vi "menuBarSelection.vi"(8 "error in (no error)":errorcluster, 10 "itemPath":string, 11 "ScriptEditorV2 in":refnum<class "ScriptEditorV2.lvclass">) -> (0 "error out":errorcluster, 2 "close":bool, 3 "ScriptEditorV2 out":refnum<class "ScriptEditorV2.lvclass">)   [LabVIEW 2009, in "Views.lvlib" / "ScriptEditor.lvlib" / "ScriptEditorV2.lvclass"]
uses:
  ScriptEditorV2.lvclass
  ScriptEditorV2.lvclass/ScriptEditorV2.ctl
  Tools/DatabaseHelpers.lvlib
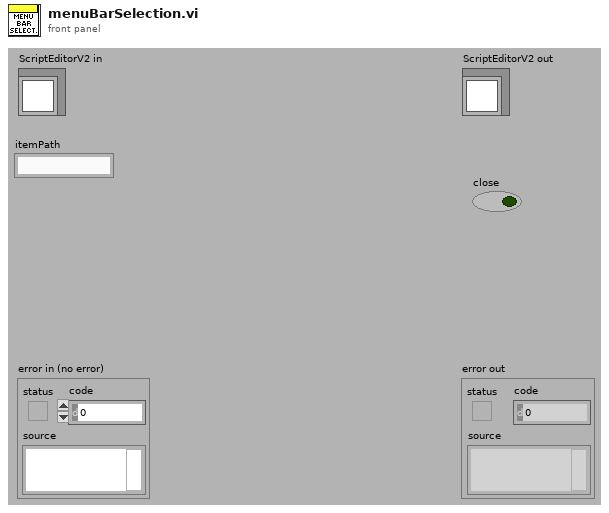
[diagram p1: front panel]
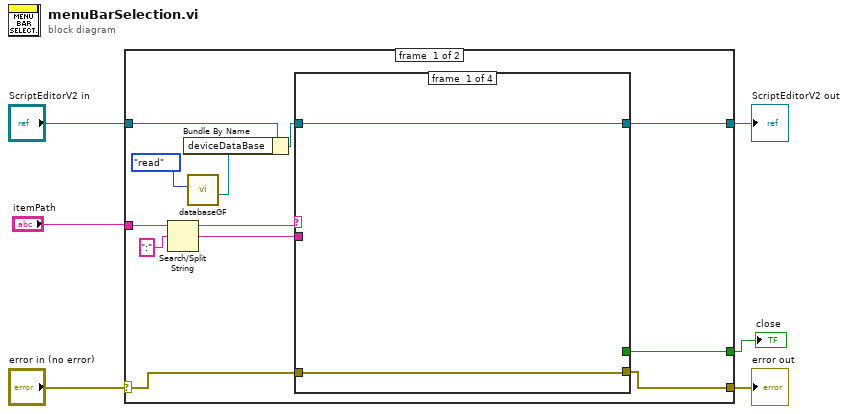
[diagram p0: block diagram]
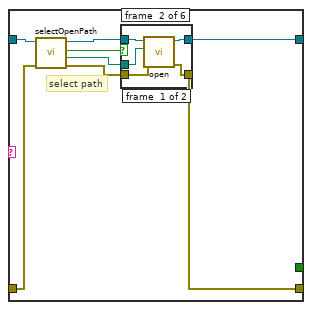
[diagram p3: hidden frame]
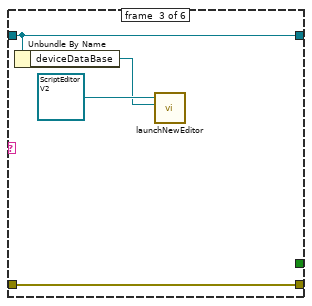
[diagram p5: hidden frame]
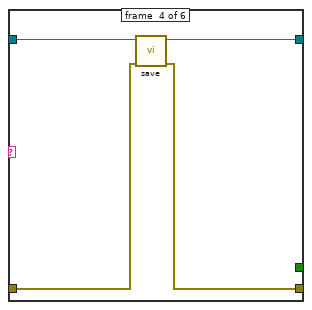
[diagram p6: hidden frame]
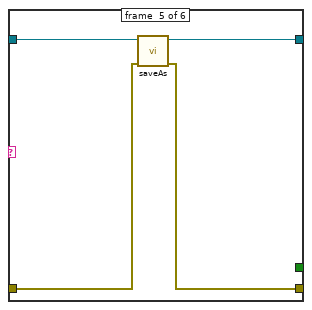
[diagram p7: hidden frame]
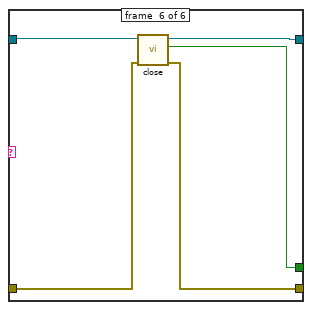
[diagram p8: hidden frame]
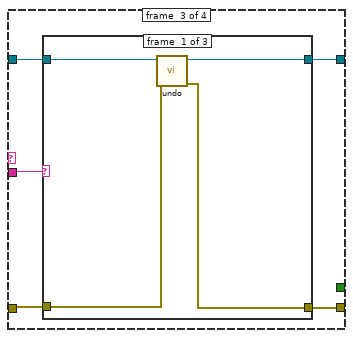
[diagram p9: hidden frame]
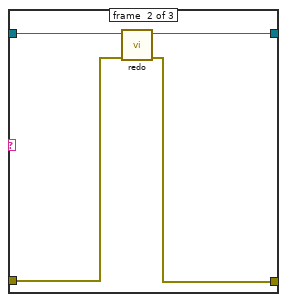
[diagram p10: hidden frame]
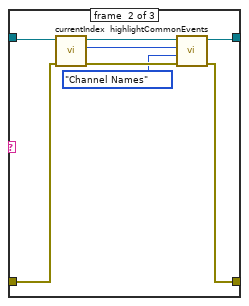
[diagram p13: hidden frame]
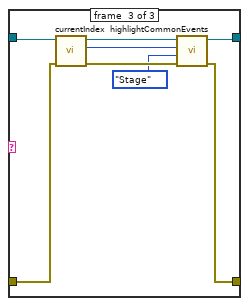
[diagram p14: hidden frame]
diagram:
  n1 = case shown="No Error" "error in (no error)" {
    selector: "error in (no error)" -> [w16 w100]
    tunnel: [w15 w100] -> w5
    tunnel: [w12 w99] -> w3
    tunnel: "ScriptEditorV2 in" -> [w8 w99]
    tunnel: "itemPath" -> [w17 _]
    tunnel: [w11 _] -> w1
    frame #0 {
      n2 = Search/Split String(string=w17, search string/char (-)=":") -> (substring before match=w14:string, match + rest of string=w13:string)  [unwired: 1 in, 1 out]
      n3 = call "databaseGF.vi"("Enum"=enum16{"write", "read"}."read") -> ("deviceDataBase out"=w9:refnum<class "deviceDataBase.lvclass">)  [unwired: 10 in]
      n4 = Bundle By Name(cluster=w8, "deviceDataBase"=w9) -> (w7:refnum<class "ScriptEditorV2.lvclass">)
      n5 = case shown="\"Edit\"" w14 {
        tunnel: w16 -> [w19 w26 w62 w77]
        tunnel: [w19 w25 w61 w76] -> w15
        tunnel: w13 -> [_ w22 w65 w78]
        tunnel: w7 -> [w20 w24 w64 w80]
        tunnel: [w20 w23 w63 w79] -> w12
        tunnel: [_ w21 _ _] -> w11
        frame #0 {
        }
        frame #1 {
          n6 = case shown="\":New\"" w22 {
            tunnel: w26 -> [w27 w29 w47 w49 w53 w58]
            tunnel: [w27 w35 w47 w48 w52 w57] -> w25
            tunnel: w24 -> [w28 w34 w45 w51 w55 w60]
            tunnel: [w28 w36 w45 w50 w54 w59] -> w23
            tunnel: [_ _ _ _ _ w56] -> w21
            frame #0 {
            }
            frame #1 {
              # "select path"
              n7 = call "selectOpenPath.vi"("error in (no error)"=w29, "ScriptEditorV2 in"=w34) -> ("error out"=w30:errorcluster, "selected path"=w32:path, "notSelected?"=w31:bool, "ScriptEditorV2 out"=w33:refnum<class "ScriptEditorV2.lvclass">)  [unwired: 6 in]
              n8 = case shown="False" w31 {
                tunnel: [w41 w43] -> w36
                tunnel: w30 -> [w40 w42]
                tunnel: [w39 w42] -> w35
                tunnel: w33 -> [w38 w43]
                tunnel: w32 -> [w37 _]
                frame #0 {
                  n9 = call "open.vi"("error in (no error)"=w40, "Path"=w37, "ScriptEditorV2 in"=w38) -> ("error out"=w39:errorcluster, "ScriptEditorV2 out"=w41:refnum<class "ScriptEditorV2.lvclass">)  [unwired: 7 in]
                }
                frame #1 {
                }
              }
            }
            frame #2 {
              n10 = Unbundle By Name(w45) -> ("deviceDataBase"=w44:refnum<class "deviceDataBase.lvclass">)
              n11 = call-dynamic "launchNewEditor.vi"("deviceDataBase"=w44, "ScriptEditorV2 in"=refnum<class "ScriptEditorV2.lvclass"> refnum ("ScriptEditorV2 in 2")) -> ()  [unwired: 8 in, 2 out]
            }
            frame #3 {
              n12 = call "save.vi"("error in (no error)"=w49, "ScriptEditorV2 in"=w51) -> ("error out"=w48:errorcluster, "ScriptEditorV2 out"=w50:refnum<class "ScriptEditorV2.lvclass">)  [unwired: 8 in]
            }
            frame #4 {
              n13 = call "saveAs.vi"("error in (no error)"=w53, "ScriptEditorV2 in"=w55) -> ("error out"=w52:errorcluster, "ScriptEditorV2 out"=w54:refnum<class "ScriptEditorV2.lvclass">)  [unwired: 8 in]
            }
            frame #5 {
              n14 = call "close.vi"("error in (no error)"=w58, "ScriptEditorV2 in"=w60) -> ("error out"=w57:errorcluster, "close"=w56:bool, "ScriptEditorV2 out"=w59:refnum<class "ScriptEditorV2.lvclass">)  [unwired: 7 in]
            }
          }
        }
        frame #2 {
          n15 = case shown="\":Undo\"" w65 {
            tunnel: w64 -> [w69 w73 w75]
            tunnel: [w68 w72 w75] -> w63
            tunnel: w62 -> [w67 w71 w74]
            tunnel: [w66 w70 w74] -> w61
            frame #0 {
              n16 = call "undo.vi"("error in (no error)"=w67, "ScriptEditorV2 in"=w69) -> ("error out"=w66:errorcluster, "ScriptEditorV2 out"=w68:refnum<class "ScriptEditorV2.lvclass">)  [unwired: 8 in]
            }
            frame #1 {
              n17 = call "redo.vi"("error in (no error)"=w71, "ScriptEditorV2 in"=w73) -> ("error out"=w70:errorcluster, "ScriptEditorV2 out"=w72:refnum<class "ScriptEditorV2.lvclass">)  [unwired: 8 in]
            }
            frame #2 {
            }
          }
        }
        frame #3 {
          n18 = case shown="\":Channel_name\"" w78 {
            tunnel: w80 -> [w82 w88 w96]
            tunnel: [w82 w90 w98] -> w79
            tunnel: w77 -> [w81 w84 w92]
            tunnel: [w81 w89 w97] -> w76
            frame #0 {
            }
            frame #1 {
              n19 = call "currentIndex.vi"("error in (no error)"=w84, "ScriptEditorV2 in"=w88) -> ("error out"=w85:errorcluster, "index"=w86:i32, "ScriptEditorV2 out"=w87:refnum<class "ScriptEditorV2.lvclass">)  [unwired: 7 in]
              n20 = call "highlightCommonEvents.vi"("error in (no error)"=w85, "Enum"=enum16{"Channel Names", "Stage"}."Channel Names", "rowIndex"=w86, "ScriptEditorV2 in"=w87) -> ("error out"=w89:errorcluster, "ScriptEditorV2 out"=w90:refnum<class "ScriptEditorV2.lvclass">)  [unwired: 6 in]
            }
            frame #2 {
              n21 = call "currentIndex.vi"("error in (no error)"=w92, "ScriptEditorV2 in"=w96) -> ("error out"=w93:errorcluster, "index"=w94:i32, "ScriptEditorV2 out"=w95:refnum<class "ScriptEditorV2.lvclass">)  [unwired: 7 in]
              n22 = call "highlightCommonEvents.vi"("error in (no error)"=w93, "Enum"=enum16{"Channel Names", "Stage"}."Stage", "rowIndex"=w94, "ScriptEditorV2 in"=w95) -> ("error out"=w97:errorcluster, "ScriptEditorV2 out"=w98:refnum<class "ScriptEditorV2.lvclass">)  [unwired: 6 in]
            }
          }
        }
      }
    }
    frame #1 {
    }
  }
  "error out" <- w5
  "ScriptEditorV2 out" <- w3
  "close" <- w1
